vi "Run2Obstacle.vi"   [LabVIEW 2016, in "Project 2 LabVIEW.lvrbt"]
uses:
  Project 2 LabVIEW.lvrbt
  <vilib>/NXT/Block Support/NXT_OutputPort.ctl
  <vilib>/NXT/LegoClasses/BrickReference/BrickReference.lvclass
  <vilib>/NXT/Subs/LVHSConnector.ctl
  <vilib>/NXT/NXTIO Xnodes/NXTIOXNode/NXTIO.xnode
  <vilib>/NXT/NXTIO Xnodes/AddressXNode/NXTIOAddress.xnode
  <vilib>/NXT/NXTIO Xnodes/NXTIONodeSubVIs/NXTMoveMotors.vi
  <vilib>/NXT/Dual Mode Library/Sensors/EV3_Ultrasonic_CM.vi
  <vilib>/NXT/Block Support/NXT_InputPort.ctl
  <vilib>/NXT/Dual Mode Library/Waits/Wait_Num(msec).vi
types:
  T1 = typedef "NXT_OutputPort.ctl" = u8
  T2 = typedef "NXT_InputPort.ctl" = u32
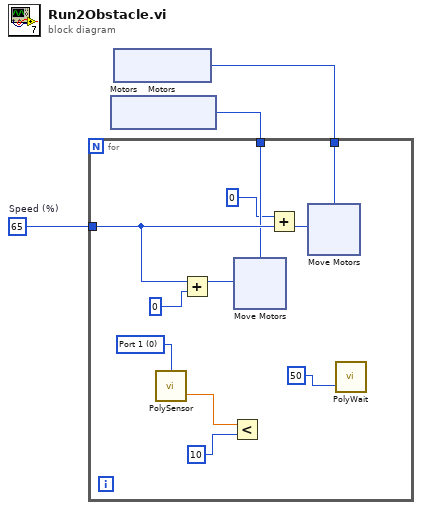
[diagram p0: block diagram]
diagram:
  w3 = 65  # Speed (%)
  n1 = xnode "Motors"() -> ("Motor"=w1:T1)
  n2 = xnode "Motors"() -> ("Motor"=w2:T1)
  n3 = for {
    tunnel: w3 -> [w14]
    tunnel: w2 -> [w10]
    tunnel: w1 -> [w9]
    w11 = T2 0 items=["Port 1", "Port 2", "Port 3", "Port 4"] ("Port (Port 1)")
    n4 = call-poly <vilib>:"PolySensor.vi"("Port (Port 1)"=w11) -> ("Centimeters"=w13:sgl)  [unwired: 2 in, 1 out]
    n5 = Add(x=w14, y=0) -> (x+y=w6:i32)
    n6 = Less?(x=w13, y=10) -> ()  [unwired: 1 out]
    n7 = xnode "Move Motors"("Power/Speed 1"=w6, "Motors"=w9) -> ()  [unwired: 1 in, 1 out]
    n8 = Add(x=0, y=w14) -> (x+y=w8:i32)
    n9 = xnode "Move Motors"("Power/Speed 1"=w8, "Motors"=w10) -> ()  [unwired: 1 in, 1 out]
    n10 = call-poly <vilib>:"PolyWait.vi"("Time (100 msec)"=50) -> ()  [unwired: 3 in, 1 out]
  }
